vi "W_open_top_levels.vi"   [LabVIEW 2021]
uses:
  ADAM Client/Sub VIs/ADAM Controls/Tunnel_speed_mode.ctl
types:
  T1 = typedef "Tunnel_speed_mode.ctl" = enum16{"Set Speed", "Set Speed then wait", "Is tunnel speed allowable?"}
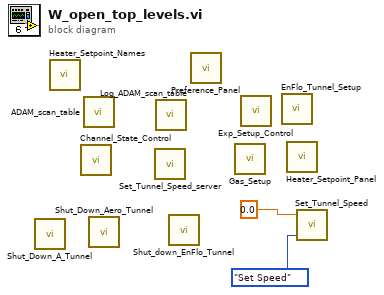
[diagram p0: block diagram]
diagram:
  n1 = call "Shut_Down_A_Tunnel.vi"() -> ()  [unwired: 3 in, 3 out]
  n2 = call "Heater_Setpoint_Names.vi"() -> ()  [unwired: 1 in, 8 out]
  n3 = call "Channel_State_Control.vi"() -> ()  [unwired: 3 in, 2 out]
  n4 = call "ADAM_scan_table.vi"() -> ()  [unwired: 4 out]
  n5 = call "Shut_Down_Aero_Tunnel.vi"() -> ()  [unwired: 3 in, 3 out]
  n6 = call "Set_Tunnel_Speed_server.vi"() -> ()  [unwired: 4 in, 4 out]
  n7 = call "Log_ADAM_scan_table.vi"() -> ()  [unwired: 5 out]
  n8 = call "Shut_down_EnFlo_Tunnel.vi"() -> ()  [unwired: 3 in, 3 out]
  n9 = call "Preference_Panel.vi"() -> ()  [unwired: 1 in]
  n10 = call "Gas_Setup.vi"() -> ()  [unwired: 9 out]
  n11 = call "Exp_Setup_Control.vi"() -> ()  [unwired: 1 in, 3 out]
  n12 = call "EnFlo_Tunnel_Setup.vi"() -> ()  [unwired: 9 out]
  n13 = call "Heater_Setpoint_Panel.vi"() -> ()  [unwired: 1 out]
  n14 = call "Set_Tunnel_Speed.vi"("Mode"=Tunnel_speed_mode."Set Speed", "Tunnel Velocity m/s"=0.0) -> ()  [unwired: 2 in, 2 out]
